vi "sedSpectrometer_monitorCommand_SetValue.vi"(8 "error in (no error)":errorcluster, 11 "command_SetValue_Ctl":T1) -> (0 "error out":errorcluster, 2 "function return":i32, 3 "command_SetValue_Ctl out":T1)   [LabVIEW 2016, in "SALLV_sedSpectrometer.lvlib"]
doc: "int sedSpectrometer_shm_monitorCommand_SetValueLV(sedSpectrometer_command_SetValueLV *command_SetValue_Ctl );"
uses:
  SALLV_sedSpectrometer.lvlib
  DataTypes/command_SetValue.ctl
  SALLV_sedSpectrometer.so
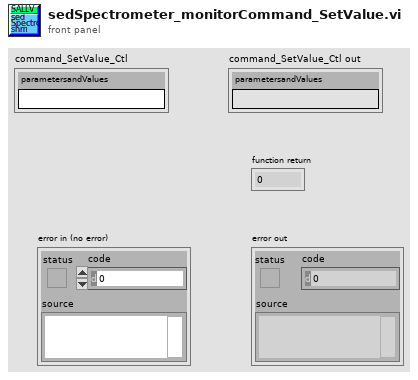
[diagram p1: front panel]
types:
  T1 = typedef "SALLV_sedSpectrometer.lvlib/command_SetValue.ctl" = cluster{"parametersandValues":string}
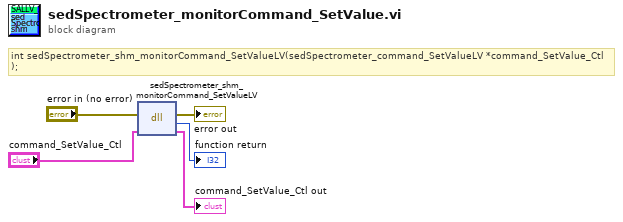
[diagram p0: block diagram]
diagram:
  # "int sedSpectrometer_shm_monitorCommand_SetValueLV(sedSpectrometer_command_SetValueLV *command_SetValue_Ctl );"
  n1 = dll-call lib="home/harini/TCS/SALLV_sedSpectrometer/SALLV_sedSpectrometer.*" fn="sedSpectrometer_shm_monitorCommand_SetValueLV"(error in="error in (no error)", "command_SetValue_Ctl"="command_SetValue_Ctl") -> (error out=→"error out":errorcluster, →"function return":i32, "command_SetValue_Ctl"=→"command_SetValue_Ctl out":T1)  [unwired: 2 in, 1 out]
